vi "Register for gRPC Server Events.vi"(8 "error in (no error)":errorcluster, 11 "CIFPlugin in":refnum<class "Template_Plugin.lvclass">) -> (0 "error out":errorcluster, 2 "Event Registration Refnum":refnum<event-registration>, 3 "CIFPlugin out":refnum<class "Template_Plugin.lvclass">)   [LabVIEW 2021, in "Template_Plugin.lvclass"]
uses:
  Template_Plugin.lvclass
  Template_Plugin.lvclass/Template_Plugin.ctl
  <vilib>/CIF Foundation/CIF Core/CIFCore/Class/CIFCorePlugin.lvclass
  Grpc/Template_server/RPC Service/Template/Template.lvclass
  <vilib>/gRPC/LabVIEW gRPC Servicer/ServiceBase/ServiceBase.lvclass
  C:/Program Files/National Instruments/LabVIEW 2021/vi.lib/CIF Foundation/CIF Core/CIFCore/Class/CIFCorePlugin.lvclass
  D:/dev/Plugins/Template/src/Source/CIF/Plugin Generator/Template/Class/Template_Plugin.lvclass
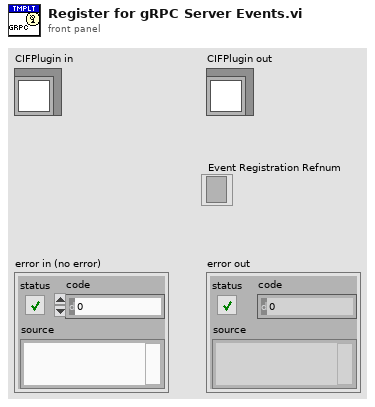
[diagram p1: front panel]
types:
  T1 = typedef "Template_server.lvlib/Template.lvclass/Server gRPC UEs.ctl" = cluster{"Template SetNumeric gRPC UE":refnum<user-event>, "Template GetResult gRPC UE":refnum<user-event>, "Template GetStatistics gRPC UE":refnum<user-event>}
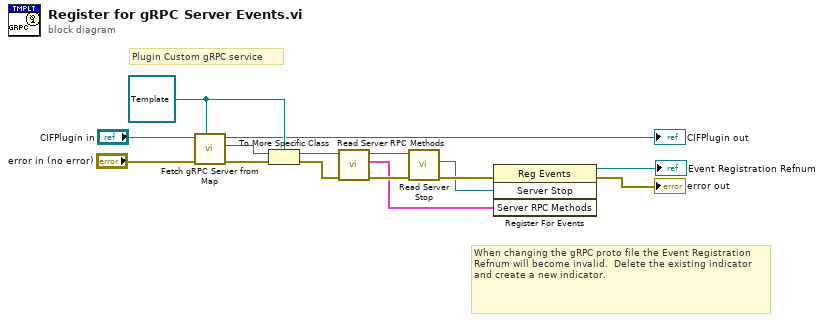
[diagram p0: block diagram]
diagram:
  w7 = refnum<class "Template.lvclass"> refnum ("CIFTemplatePlugin_server.lvlib:TemplatePlugin.lvclass")
  # "When changing the gRPC proto file the Event Registration Refnum will become invalid.  Delete the existing indicator and create a new indicator."
  # "Plugin Custom gRPC service"
  n1 = call <vilib>:"Fetch gRPC Server from Map.vi"("gRPC Server Class type"=w7, "error in (no error)"="error in (no error)", "CIFCorePlugin in"="CIFPlugin in") -> ("error out"=w11:errorcluster, "gRPC Server Class out"=w10:refnum<class "ServiceBase.lvclass">, "CIFCorePlugin out"=→"CIFPlugin out":refnum<class "Template_Plugin.lvclass">)  [unwired: 6 in]
  n2 = To More Specific Class(target class=w7, reference=w10, error in=w11) -> (specific class reference=w12:refnum<class "Template.lvclass">, error out=w6:errorcluster)
  n3 = call "Read Server RPC Methods.vi"("error in (no error)"=w6, "SignalGeneratorService in"=w12) -> ("error out"=w13:errorcluster, "Server RPC Methods"=w3:T1, "SignalGeneratorService out"=w14:refnum<class "Template.lvclass">)  [unwired: 7 in]
  n4 = call-dynamic "Read Server Stop.vi"("error in"=w13, "iService in"=w14) -> ("error out"=w4:errorcluster, "Server Stop"=w2:refnum<user-event>)  [unwired: 7 in, 1 out]
  n5 = register-events(error in=w4, w2, w3) -> (reference out=→"Event Registration Refnum":refnum<event-registration>, error out=→"error out":errorcluster)  [unwired: 1 in]
